vi "HTTP Communication.vi"(8 "error in":errorcluster, 10 "Cameras Enabled":cluster{"rgb_camera":bool, "hsi_camera":bool}={"rgb_camera"=TRUE, "hsi_camera"=TRUE}, 11 "Data":T1={"HTTP Queue"=refnum, "Notifier"=refnum, "Photo Save Directory"=path "", "Photo Period (ms)"=0, "Cameras Enabled"={"rgb_camera"=TRUE, "hsi_camera"=TRUE}, "Config ID"=0}) -> (0 "error out":errorcluster)   [LabVIEW 2023]
doc: "Main VI for HTTP communication."
uses:
  <vilib>/ErrorRing/Error Ring.xnode
  <vilib>/httpClient/LabVIEWHTTPClient.lvlib
  <vilib>/httpClient/POSTBuffer.vi
  <vilib>/Utility/error.llb/Error Cluster From Error Code.vi
  <vilib>/numeric/Random Number (Range) U64.vi
  defs/HTTP Queue Definition.ctl
  defs/Notification Definition.ctl
  defs/Data.ctl
panel:
  in  "Stop":bool
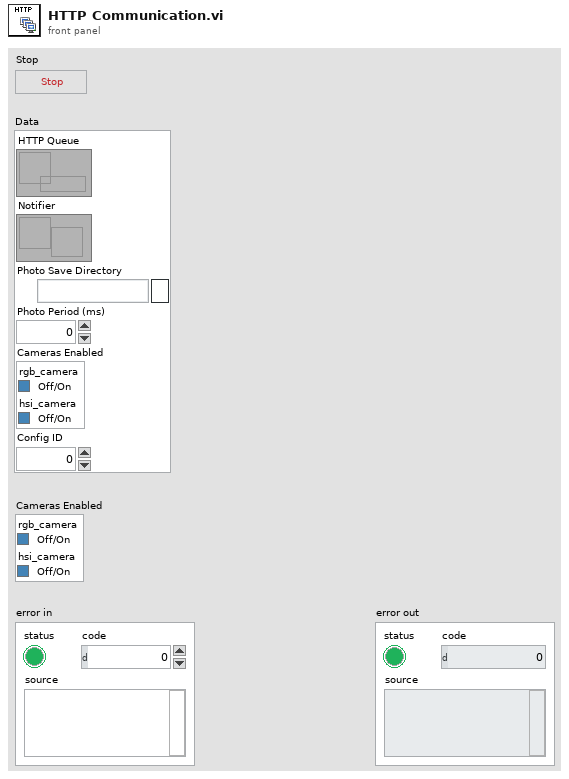
[diagram p1: front panel]
types:
  T1 = typedef "Data.ctl" = cluster{"HTTP Queue":refnum<queue>, "Notifier":refnum<notifier>, "Photo Save Directory":path, "Photo Period (ms)":u32, "Cameras Enabled":cluster{"rgb_camera":bool, "hsi_camera":bool}, "Config ID":u32}
  T2 = typedef "LabVIEWHTTPClient.lvlib/ClientHandle.ctl" = refnum<k1>
  T3 = typedef "HTTP Queue Definition.ctl" = cluster{"Message":string, "Photo Path":path}
  T4 = typedef "Notification Definition.ctl" = cluster{"Message":string}
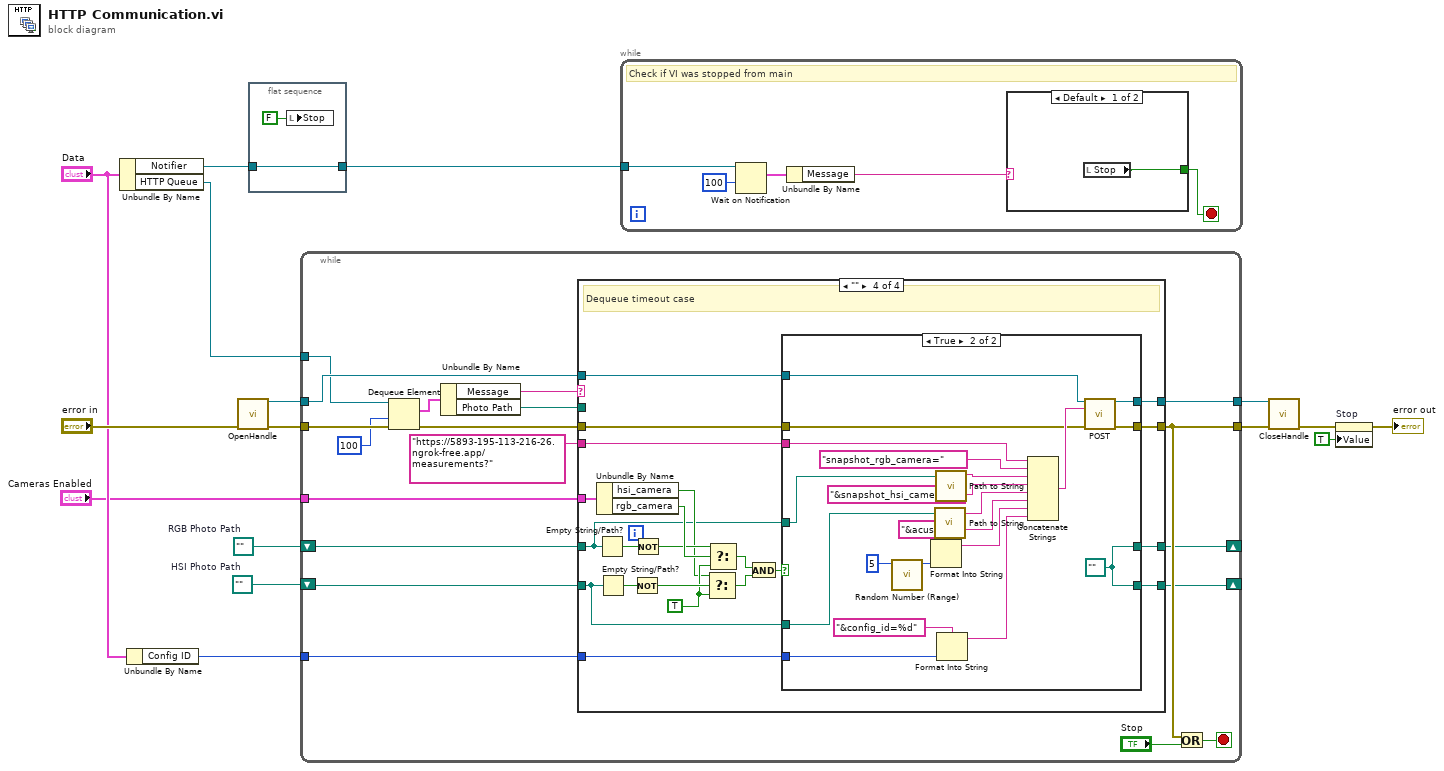
[diagram p0: block diagram]
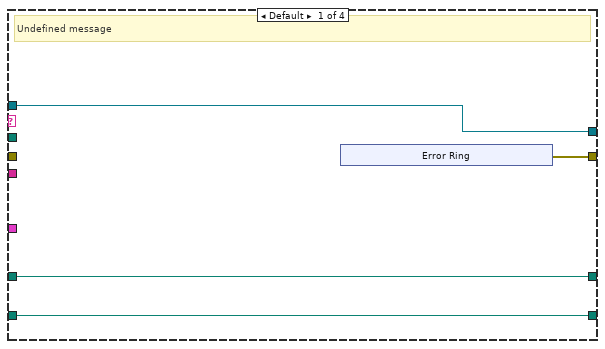
[diagram p2: hidden frame]
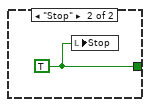
[diagram p6: hidden frame]
diagram:
  w2 = path ""  # HSI Photo Path
  w3 = path ""  # RGB Photo Path
  n1 = Unbundle By Name("Data") -> ("Notifier"=w7:refnum<notifier>, "HTTP Queue"=w6:refnum<queue>)
  n2 = Unbundle By Name("Data") -> ("Config ID"=w4:u32)
  n3 = call <vilib>:"OpenHandle.vi"("error in (no error)"="error in") -> ("client handle out"=w15:T2, "error out"=w14:errorcluster)  [unwired: 13 in]
  n4 = flat-sequence {
    tunnel: w7 -> [w17]
    tunnel: [w17] -> w8
    frame #0 {
      n5 = local write "Stop"(FALSE ("Stop")) -> ()
    }
  }
  n6 = while {
    tunnel: w15 -> [w34]
    tunnel: [w37] -> w13
    tunnel: w6 -> [w33]
    tunnel: w14 -> [w36]
    tunnel: [w28] -> w12
    tunnel: w4 -> [w25]
    shift-right: [w22] -> _
    shift-left: w3 -> [w23]
    shift-right: [w21] -> _
    shift-left: w2 -> [w20]
    tunnel: "Cameras Enabled" -> [w19]
    stop <- w29 stop-if-true
    n7 = Dequeue Element(queue=w33, timeout in ms (-1)=100, error in (no error)=w36) -> (element=w32:T3, error out=w35:errorcluster)  [unwired: 2 out]
    n8 = Unbundle By Name(w32) -> ("Message"=w31:string, "Photo Path"=w30:path)
    n9 = case shown="\"\"" w31 {
      tunnel: w34 -> [w40 w46 w53 w61]
      tunnel: w35 -> [_ w47 w52 w62]
      tunnel: [w40 w46 w53 w60] -> w37
      tunnel: [w41 w47 w52 w59] -> w28
      tunnel: w30 -> [_ w49 w51 _]
      tunnel: w25 -> [_ _ _ w58]
      tunnel: "https://5893-195-113-216-26.ngrok-free.app/measurements?" ("url") -> [_ _ _ w63]
      tunnel: w23 -> [w39 w48 _ w57]
      tunnel: [w39 w48 w51 w55] -> w22
      tunnel: [w38 w49 w50 w54] -> w21
      tunnel: w20 -> [w38 _ w50 w56]
      tunnel: w19 -> [_ _ _ w74]
      frame Default {
        # "Undefined message"
        n10 = xnode "Error Ring"() -> ("error out"=w41:errorcluster)
      }
      frame "Hyperspectral Photo Taken" {
        # "Send POST that hyperspectral photo was taken"
      }
      frame "RGB Photo Taken" {
        # "Send POST that RGB photo was taken"
      }
      frame "" {
        w68 = TRUE ("f")
        # "Dequeue timeout case"
        n11 = Unbundle By Name(w74) -> ("hsi_camera"=w67:bool, "rgb_camera"=w71:bool)
        n12 = Empty String/Path?(string/path=w57) -> (empty?=w72:bool)
        n13 = Empty String/Path?(string/path=w56) -> (empty?=w73:bool)
        n14 = Not(x=w73) -> (.not. x?=w69:bool)
        n15 = Not(x=w72) -> (.not. x?=w70:bool)
        n16 = Select(t=w67, s=w69, f=w68) -> (s? t:f=w66:bool)
        n17 = Select(t=w70, s=w71, f=w68) -> (s? t:f=w65:bool)
        n18 = And(x=w65, y=w66) -> (x .and. y?=w64:bool)
        n19 = case shown="True" w64 {
          tunnel: w63 -> [_ w94]
          tunnel: w62 -> [w78 w93]
          tunnel: w61 -> [w77 w92]
          tunnel: [w77 w91] -> w60
          tunnel: [w78 w90] -> w59
          tunnel: w58 -> [_ w89]
          tunnel: w57 -> [w76 w82]
          tunnel: w56 -> [w75 w80]
          tunnel: [w76 w83] -> w55
          tunnel: [w75 w83] -> w54
          frame False {
          }
          frame True {
            w83 = path ""
            n20 = call-poly <vilib>:"Random Number (Range).vi"("upper bound (100)"=u64 5) -> ("number"=w97:u64)  [unwired: 10 in]
            n21 = Format Into String(w97) -> (resulting string=w87:string)  [unwired: 3 in, 1 out]
            n22 = call "Path to String.vi"("Path In"=w80) -> ("Path String"=w79:string)  [unwired: 10 in]
            n23 = call "Path to String.vi"("Path In"=w82) -> ("Path String"=w81:string)  [unwired: 10 in]
            n24 = Format Into String(format string="&config_id=%d" ("string"), w89) -> (resulting string=w88:string)  [unwired: 2 in, 1 out]
            n25 = Concatenate Strings(w94, "snapshot_rgb_camera=" ("url"), w81, "&snapshot_hsi_camera=" ("string"), w79, "&acustic=" ("string"), w87, w88) -> (w96:string)
            n26 = call-poly <vilib>:"POST.vi"("client handle"=w92, "url"=w96, "error in (no error)"=w93) -> ("client handle out"=w91:T2, "error out"=w90:errorcluster)  [unwired: 9 in, 2 out]
          }
        }
      }
    }
    n27 = Or(x=w28, y="Stop") -> (x .or. y?=w29:bool)
  }
  n28 = while {
    tunnel: w8 -> [w103]
    stop <- w100 stop-if-true
    # "Check if VI was stopped from main"
    n29 = Wait on Notification(notifier=w103, timeout in ms (-1)=100) -> (notification=w102:T4)  [unwired: 2 in, 3 out]
    n30 = Unbundle By Name(w102) -> ("Message"=w101:string)
    n31 = case shown="Default" w101 {
      tunnel: [w104 w105] -> w100
      frame Default {
        n32 = local read "Stop"() -> (w104:bool)
      }
      frame "Stop" {
        w105 = TRUE
        n33 = local write "Stop"(w105) -> ()
      }
    }
  }
  n34 = call <vilib>:"CloseHandle.vi"("client handle"=w13, "error in (no error)"=w12) -> ("error out"=w11:errorcluster)  [unwired: 13 in]
  n35 = property on="Stop" class="Bool (strict)"(error in=w11, "Value"=TRUE ("Stop")) -> (error out=→"error out":errorcluster)  [unwired: 1 in, 1 out]
